vi "HWLV6.vi"() -> ()   [LabVIEW 2023]
panel:
  out "Waveform Chart":dbl(graph)
  in  "Z":dbl
  in  "Y":dbl
  in  "X":dbl
  in  "Number of iterations":dbl
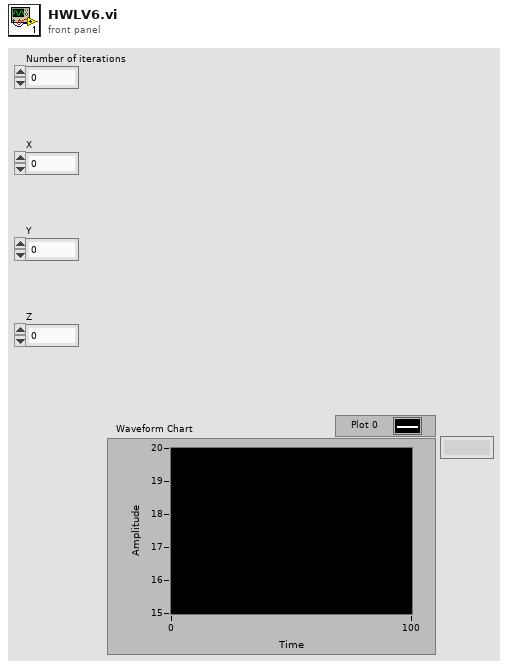
[diagram p1: front panel]
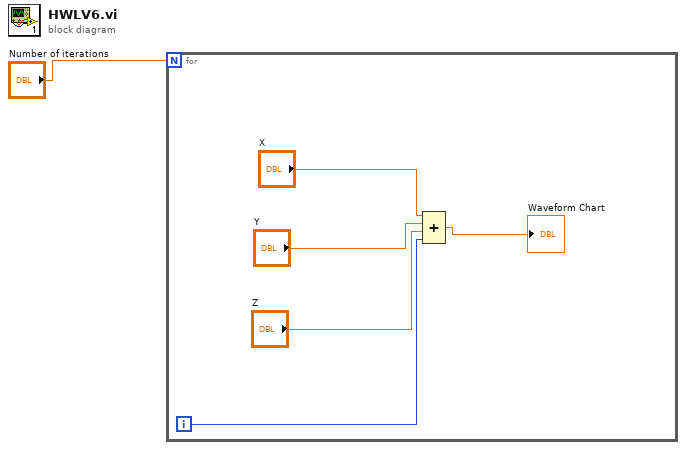
[diagram p0: block diagram]
diagram:
  n1 = for {
    N: "Number of iterations" -> [_]
    i -> [w3]
    n2 = Compound Arithmetic op=ADD("X", "Y", "Z", w3) -> (→"Waveform Chart":dbl)
  }
